vi "get previous sample.vi"(8 "error in (no error)":errorcluster, 11 "Automation in":refnum<class "Automation.lvclass">) -> (0 "error out":errorcluster, 1 "Polarization":dbl, 2 "Eventnum":i64, 3 "Automation out":refnum<class "Automation.lvclass">)   [LabVIEW 2019, in "Automation.lvclass"]
uses:
  Automation.lvclass
  Automation.lvclass/Automation.ctl
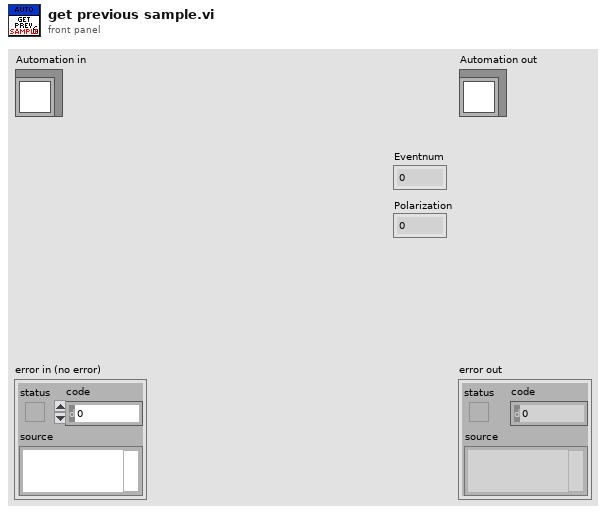
[diagram p1: front panel]
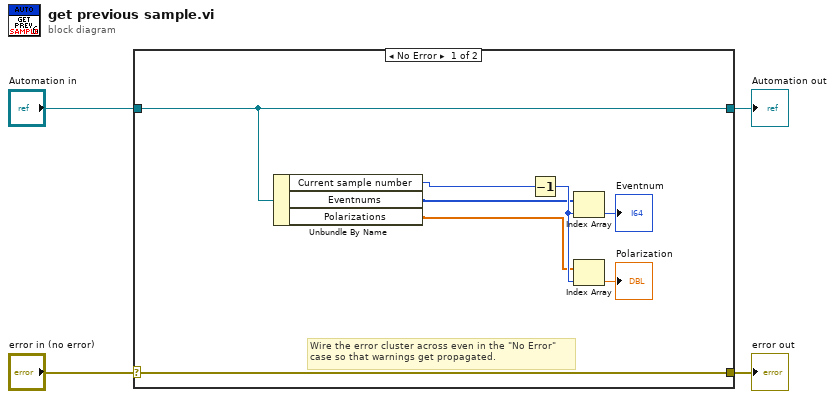
[diagram p0: block diagram]
diagram:
  n1 = case shown="No Error" "error in (no error)" {
    selector: "error in (no error)" -> [w12 w14]
    tunnel: [w12 w14] -> w3
    tunnel: [w11 w13] -> w1
    tunnel: "Automation in" -> [w11 w13]
    frame No Error {
      # "Wire the error cluster across even in the \"No Error\"\ncase so that warnings get propagated."
      n2 = Unbundle By Name(w11) -> ("Current sample number"=w7:i32, "Eventnums"=w6:i64[], "Polarizations"=w5:dbl[])
      n3 = Decrement(x=w7) -> (x-1=w10:i32)
      n4 = Index Array(array=w6, index=w10) -> (element=→"Eventnum":i64)
      n5 = Index Array(array=w5, index=w10) -> (element=→"Polarization":dbl)
    }
    frame Error {
    }
  }
  "error out" <- w3
  "Automation out" <- w1
